vi "read_params.vi"(8 "error in (no error)":errorcluster, 11 "LocallyLinearEmbedding in":refnum<class "LocallyLinearEmbedding.lvclass">) -> (0 "error out":errorcluster, 2 "params":T1={"n_neighbors"=5.0, "n_components"=2.0, "reg"=0.001, "eigen_solver"="auto", "tol"=1e-06, "max_iter"=100.0, "method"="standard", "hessian_tol"=0.0001, "modified_tol"=1e-12, "neighbors_algorithm"="auto", "random_state"=0.0, "n_jobs"=1.0}, 3 "LocallyLinearEmbedding out":refnum<class "LocallyLinearEmbedding.lvclass">)   [LabVIEW 2020, in "LocallyLinearEmbedding.lvclass"]
uses:
  LocallyLinearEmbedding.lvclass
  Controls/locally_linear_embedding_params.ctl
  LocallyLinearEmbedding.lvclass/LocallyLinearEmbedding.ctl
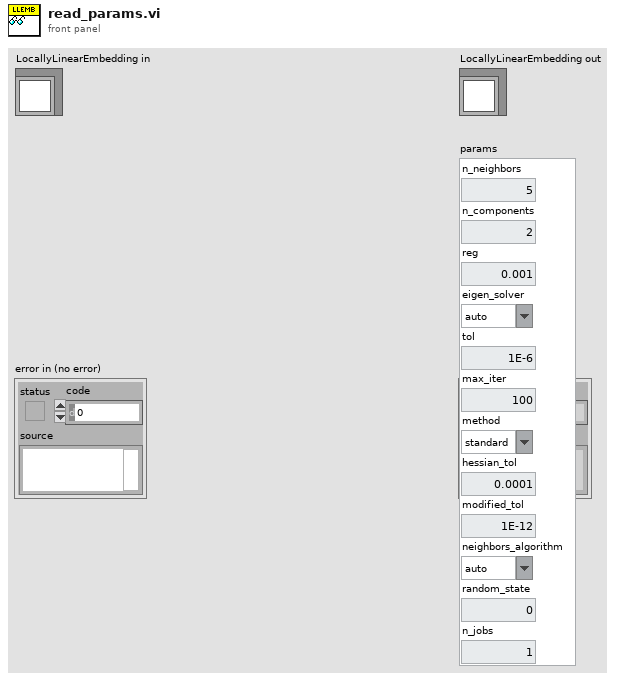
[diagram p1: front panel]
types:
  T1 = typedef "locally_linear_embedding_params.ctl" = cluster{"n_neighbors":dbl, "n_components":dbl, "reg":dbl, "eigen_solver":string, "tol":dbl, "max_iter":dbl, "method":string, "hessian_tol":dbl, "modified_tol":dbl, "neighbors_algorithm":string, "random_state":dbl, "n_jobs":dbl}
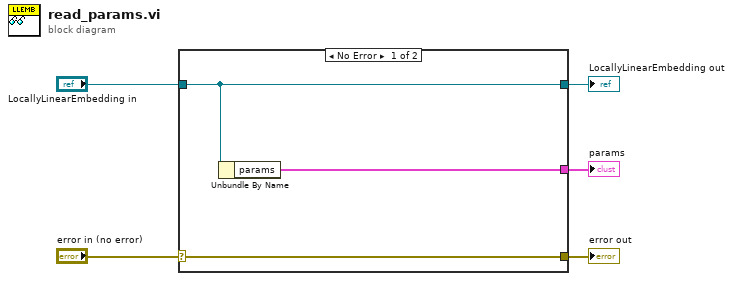
[diagram p0: block diagram]
diagram:
  n1 = case shown="No Error" "error in (no error)" {
    selector: "error in (no error)" -> [w8 w9]
    tunnel: [w8 w9] -> w4
    tunnel: [w7 w10] -> w2
    tunnel: "LocallyLinearEmbedding in" -> [w7 w10]
    tunnel: [w6 _] -> w1
    frame No Error {
      n2 = Unbundle By Name(w7) -> ("params"=w6:T1)
    }
    frame Error {
    }
  }
  "error out" <- w4
  "LocallyLinearEmbedding out" <- w2
  "params" <- w1
